vi "Get Frame-Owner Array.vi"(9 "Diagram out":refnum<vi>, 11 "References":refnum<vi>[](array[refnum])) -> (3 "Frames-Owners":T1(array[cluster]))   [LabVIEW 2026]
doc: "This vi accepts a reference to a block diagram and an array of structure names. It loops through all instances of those structures found in the diagram, and returns an array of references to every possible frame in that diagram, each paired with a reference to its owner and the class name of the structure."
panel:
  out "Diagram in":refnum<vi>
  # "GObject"
  # "Owner"
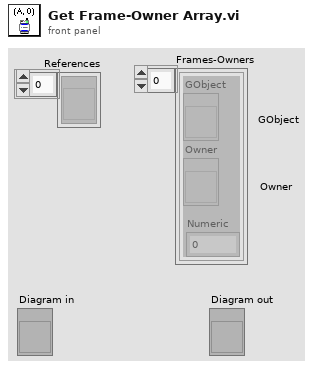
[diagram p1: front panel]
types:
  T1 = cluster{"GObject":refnum<vi>, "Owner":refnum<vi>, "Numeric":dbl}[]
  T2 = cluster{refnum<vi>, "Owner":refnum<vi>, "UID":i32}
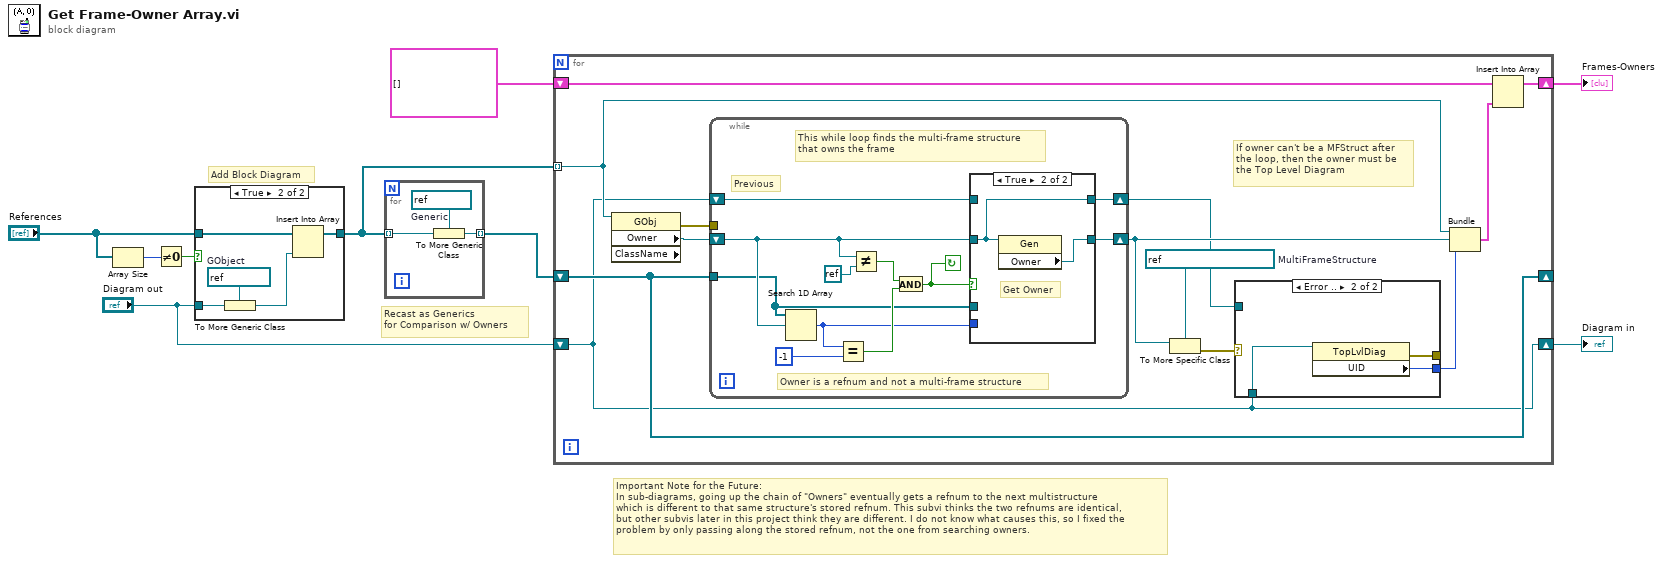
[diagram p0: block diagram]
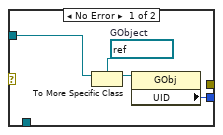
[diagram p3: hidden frame]
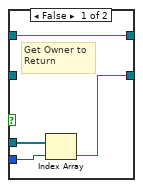
[diagram p4: hidden frame]
diagram:
  # "Recast as Generics\nfor Comparison w/ Owners"
  # "Add Block Diagram"
  # "Important Note for the Future:\nIn sub-diagrams, going up the chain of \"Owners\" eventually gets a refnum to the next multistructure\nwhich is different to that same structure's stored refnum. This subvi thinks the two refnums are identical,\nbut other subvis later in this project think they are different. I do not know what causes this, so I fixed the\nproblem by only passing along the stored refnum, not the one from searching owners."
  n1 = Array Size(array="References") -> (size(s)=w5:i32)
  n2 = Not Equal To 0?(x=w5) -> (x != 0?=w6:bool)
  n3 = case shown="True" w6 {
    tunnel: "References" -> [w10 w15]
    tunnel: "Diagram out" -> [_ w13]
    tunnel: [w10 w14] -> w4
    frame False {
    }
    frame True {
      w12 = refnum<vi> refnum  # GObject
      n4 = To More Generic Class(target class=w12, reference=w13) -> (generic class reference=w11:refnum<vi>)
      n5 = Insert Into Array(array=w15, new element=w11) -> (w14:refnum<vi>[])  [unwired: 1 in]
    }
  }
  n6 = for {
    tunnel: w4 -> [w16] mode=indexing
    tunnel: [w18] -> w9 mode=indexing
    w17 = refnum<vi> refnum  # Generic
    n7 = To More Generic Class(target class=w17, reference=w16) -> (generic class reference=w18:refnum<vi>)
  }
  n8 = for {
    shift-right: [w31] -> _
    shift-left: w9 -> [w31]
    shift-right: [w29] -> w7
    shift-left: cluster{refnum<vi>, "Owner":refnum<vi>, i32}[] [] -> [w30]
    tunnel: w4 -> [w23] mode=indexing
    shift-right: [w20] -> w1
    shift-left: "Diagram out" -> [w20]
    w26 = refnum<vi> refnum  # MultiFrameStructure
    # "If owner can't be a MFStruct after\nthe loop, then the owner must be\nthe Top Level Diagram"
    n9 = property class="GObj" props=["Owner", "ClassName"](reference=w23) -> (error out=w19:errorcluster, "Owner"=w28:refnum<vi>)  [unwired: 1 in, 2 out]
    n10 = while {
      shift-right: [w49] -> w22
      shift-left: w28 -> [w43]
      tunnel: w31 -> [w41]
      shift-right: [w40] -> w21
      shift-left: w20 -> [w39]
      tunnel: w19 -> [_]
      stop <- w44 continue-if-true
      # "This while loop finds the multi-frame structure\nthat owns the frame"
      # "Owner is a refnum and not a multi-frame structure"
      # "Previous"
      n11 = Search 1D Array(1D array=w41, element=w43) -> (index of element=w42:i32)  [unwired: 1 in]
      n12 = Equal?(x=w42, y=-1) -> (x = y?=w45:bool)
      n13 = Not Equal?(x=w43, y=refnum<k0> refnum) -> (x != y?=w47:bool)
      n14 = And(x=w47, y=w45) -> (x .and. y?=w44:bool)
      n15 = case shown="True" w44 {
        tunnel: w43 -> [_ w54]
        tunnel: [w51 w55] -> w49
        tunnel: w42 -> [w53 _]
        tunnel: w41 -> [w52 _]
        tunnel: [w50 w54] -> w40
        tunnel: w39 -> [w50 _]
        frame False {
          # "Get Owner to\nReturn"
          n16 = Index Array(array=w52, index=w53) -> (element=w51:refnum<vi>)
        }
        frame True {
          # "Get Owner"
          n17 = property class="Gen"(reference=w54) -> ("Owner"=w55:refnum<vi>)  [unwired: 1 in, 2 out]
        }
      }
    }
    n18 = To More Specific Class(target class=w26, reference=w22) -> (error out=w25:errorcluster)  [unwired: 1 in, 1 out]
    n19 = case shown="Error .." w25 {
      tunnel: [w32 w38] -> w24
      tunnel: w21 -> [w35 _]
      tunnel: w20 -> [_ w37]
      tunnel: [_ w36] -> _
      frame No Error {
        w34 = refnum<vi> refnum  # GObject
        n20 = To More Specific Class(target class=w34, reference=w35) -> (specific class reference=w33:refnum<vi>)  [unwired: 1 in, 1 out]
        n21 = property class="GObj"(reference=w33) -> ("UID"=w32:i32)  [unwired: 1 in, 2 out]
      }
      frame Error {
        n22 = property class="TopLvlDiag"(reference=w37) -> (error out=w36:errorcluster, "UID"=w38:i32)  [unwired: 1 in, 1 out]
      }
    }
    n23 = Bundle(w23, "Owner"=w22, "UID"=w24) -> (w27:T2)  [unwired: 1 in]
    n24 = Insert Into Array(array=w30, new element=w27) -> (w29:cluster{refnum<vi>, "Owner":refnum<vi>, i32}[])  [unwired: 1 in]
  }
  "Frames-Owners" <- w7
  "Diagram in" <- w1
